vi "Hemolymph.vi"() -> ()   [LabVIEW 2017]
uses:
  <vilib>/vision/NI_Vision_Development_Module.lvlib
panel:
  in  "Tab Control":enum32{"Parameters", "Data"}(tab)
  in  "End":dbl
  in  "Start":dbl
  in  "FPS":dbl
  in  "JPG or AVI":bool
  in  "Frame":i32(slide) min=0 max=10556 step=1 scale=0.0..10556.0
  out "Original":T1(plugin-control)
  in  "Stop Button":bool
  in  "Parameters":T2={"Look for"=0, "Window Size(32x32)"={"SizeX"=32, "SizeY"=32}, "Niblack Deviation Factor"=0.2, "Range"={"Lower value"=128, "Upper value"=255}, "Number of Erosion"=2} {"Range"."Upper value" scale=0.0..255.0; "Range"."Lower value" scale=0.0..255.0; "Niblack Deviation Factor" min=0.0 max=1.0 format="%.2f"; "Window Size(32x32)"."SizeY" min=3 step=1; "Window Size(32x32)"."SizeX" min=3 step=1; "Look for" items=["Bright Objects", "Dark Objects"]}
  in  "Method":i32(ring) items=["Niblack", "Background Correction", "Constant Threshold", "Auto Threshold"]
  out "Threshold":T1(plugin-control)
  out "Improved Threshold":T1(plugin-control)
  out "Clamped":T1(plugin-control)
  in  "Extract Length":bool
  out "Time":dbl[](array[numeric])
  out "Number of frames":dbl
  in  "Fit Length":bool
  out "Velocity":cluster{"Time":dbl[], dbl[]}(graph)
  out "Length":cluster{dbl[], sgl[]}(graph)
  out "Fit":cluster{"Time":dbl[], "mean":dbl[]}[](graph)
  in  "No of Avg":i32
  out "Distance":sgl[](array[numeric]) format="%.2f"
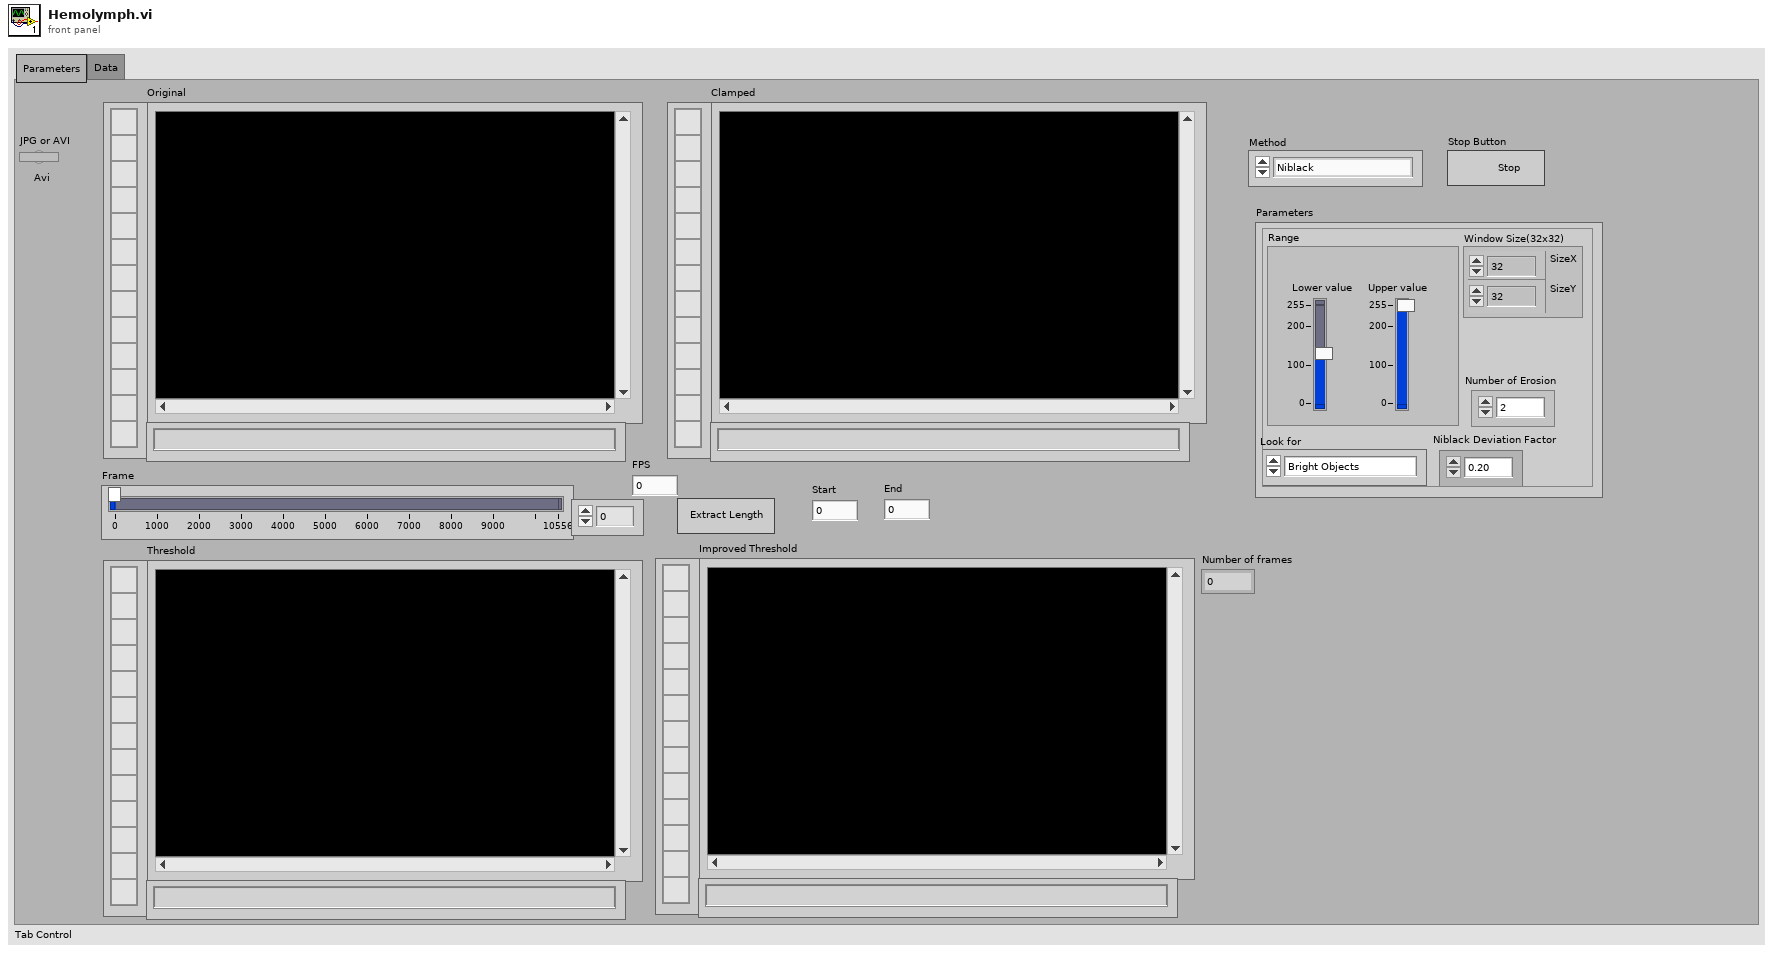
[diagram p1: front panel]
types:
  T1 = typedef "IMAQ Image.ctl" = refnum<image>
  T2 = cluster{"Look for":i32, "Window Size(32x32)":cluster{"SizeX":i32, "SizeY":i32}, "Niblack Deviation Factor":dbl, "Range":cluster{"Lower value":i32, "Upper value":i32}, "Number of Erosion":i32}
  T3 = cluster{"Global Rectangle":i32[], "Contours":cluster{"Contour Type":u32, "ROI Type":u32, "Points":i32[]}[]}
  T4 = typedef "IMAQ Rectangle" = cluster{"Left":i32, "Top":i32, "Right":i32, "Bottom":i32, "Rotation":dbl}
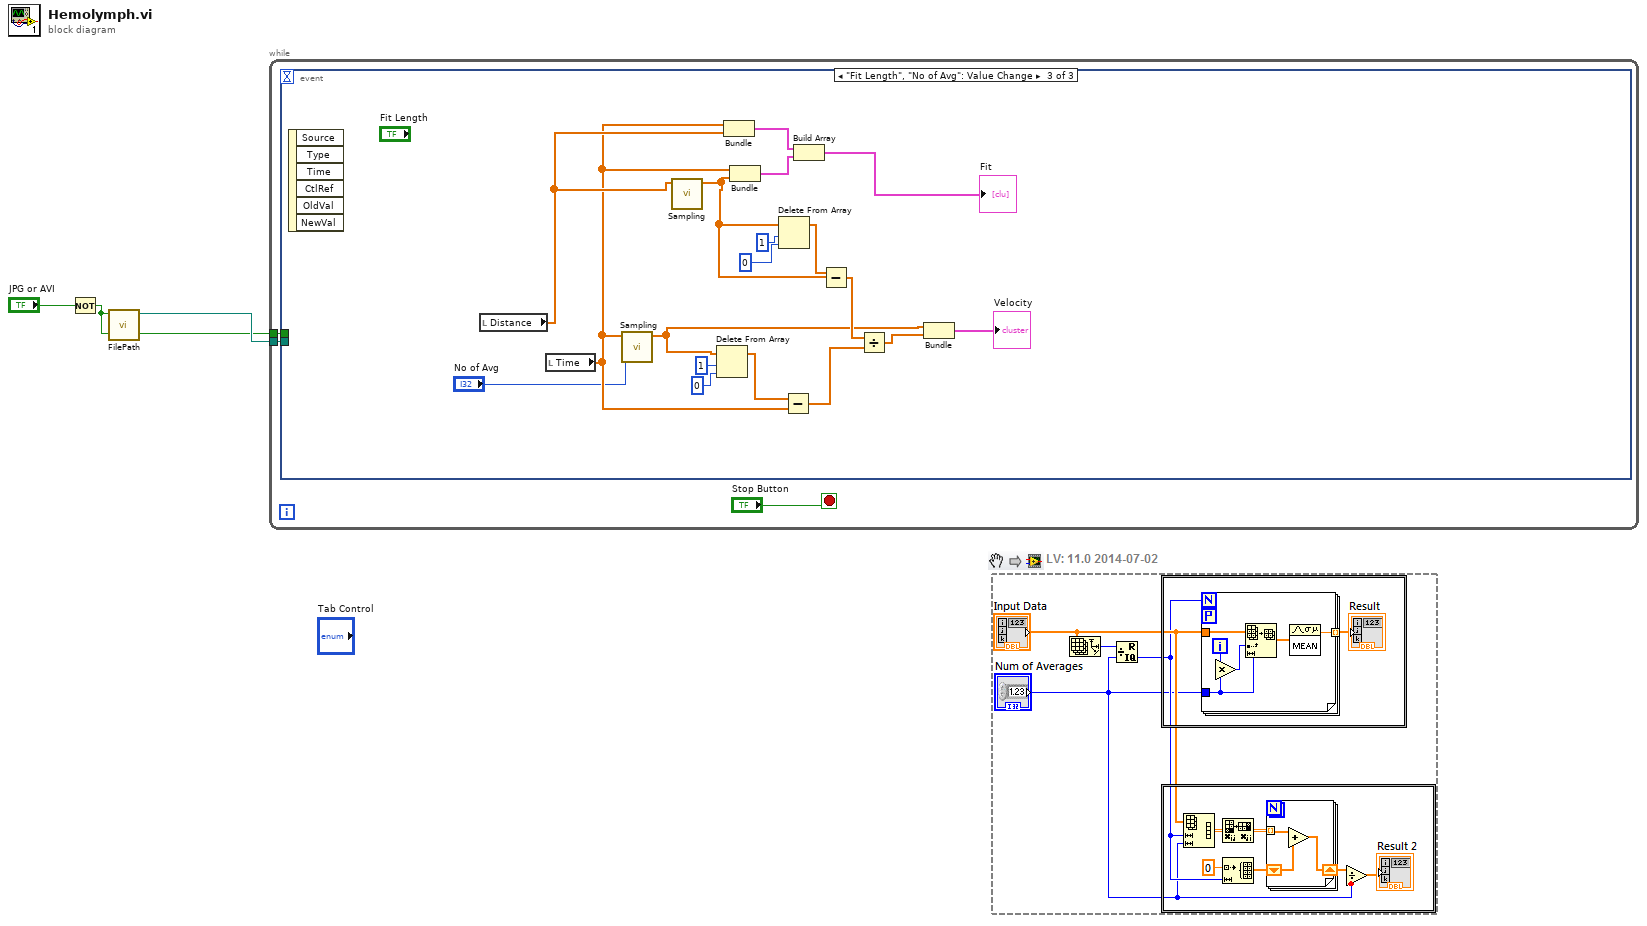
[diagram p0: block diagram]
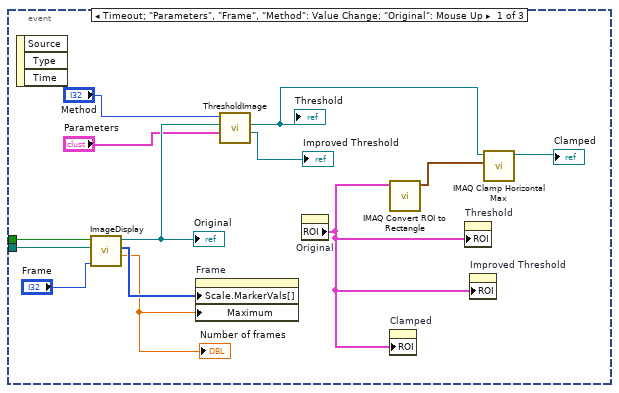
[diagram p2: hidden frame]
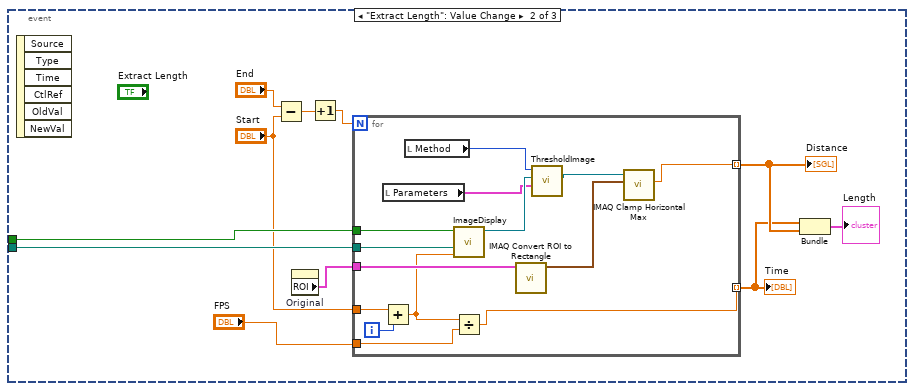
[diagram p3: hidden frame]
diagram:
  n1 = Not(x="JPG or AVI") -> (.not. x?=w1:bool)
  n2 = call "FilePath.vi"("Boolean"=w1) -> ("Path"=w3:path)  [unwired: 10 in]
  n3 = while {
    tunnel: w3 -> [w6]
    tunnel: w1 -> [w5]
    stop <- "Stop Button" stop-if-true
    n4 = event shown="[2] \"Fit Length\", \"No of Avg\": Value Change" {
      selector: _ -> [_ _ _]
      dyn-events: _ -> [_ _ _]
      timeout: _ -> [_ _ _]
      tunnel: w6 -> [w19 w29 _]
      tunnel: w5 -> [w17 w30 _]
      event Timeout; "Parameters", "Frame", "Method": Value Change; "Original": Mouse Up {
        n5 = event-data() -> ()  [unwired: 1 in, 3 out]
        n6 = call "ImageDisplay.vi"("Frame"="Frame", "Path"=w19, "JPG or AVI"=w17) -> ("Number of frames"=w15:dbl, "Frames"=w16:u32[], "Image"=w14:T1)  [unwired: 5 in]
        "Original" <- w14
        "Number of frames" <- w15
        n7 = property on="Frame" class="Slide (strict)"("Scale.MarkerVals[]"=w16, "Maximum"=w15) -> ()  [unwired: 2 in, 2 out]
        n8 = call "ThresholdImage.vi"("Method"="Method", "Image Src"=w14, "Cluster"="Parameters") -> ("Threshold"=w9:T1, "Improved Threshold"=→"Improved Threshold":T1)  [unwired: 6 in]
        "Threshold" <- w9
        n9 = property on="Original" class="ImageControl"() -> ("ROI"=w7:T3)  [unwired: 2 in, 2 out]
        n10 = call "IMAQ Convert ROI to Rectangle"("ROI Descriptor"=w7) -> ("Rectangle"=w10:T4)  [unwired: 8 in, 1 out]
        n11 = property on="Clamped" class="ImageControl"("ROI"=w7) -> ()  [unwired: 2 in, 2 out]
        n12 = property on="Threshold" class="ImageControl"("ROI"=w7) -> ()  [unwired: 2 in, 2 out]
        n13 = property on="Improved Threshold" class="ImageControl"("ROI"=w7) -> ()  [unwired: 2 in, 2 out]
        n14 = call "IMAQ Clamp Horizontal Max"("Rectangle"=w10, "Image"=w9) -> ("Image Out"=→"Clamped":T1)  [unwired: 5 in, 4 out]
      }
      event "Extract Length": Value Change {
        n15 = event-data() -> ()  [unwired: 1 in, 6 out]
        n16 = Subtract(x="End", y="Start") -> (x-y=w25:dbl)
        n17 = property on="Original" class="ImageControl"() -> ("ROI"=w28:T3)  [unwired: 2 in, 2 out]
        n18 = Increment(x=w25) -> (x+1=w24:dbl)
        n19 = for {
          N: w24 -> [_]
          tunnel: w30 -> [w44]
          tunnel: w29 -> [w43]
          tunnel: [w42] -> w21 mode=indexing
          tunnel: w28 -> [w41]
          tunnel: [w39] -> w22 mode=indexing
          tunnel: "FPS" -> [w34]
          tunnel: "Start" -> [w31]
          i -> [w33]
          n20 = local read "Parameters"() -> (w36:T2)
          n21 = Add(x=w31, y=w33) -> (x+y=w32:dbl)
          n22 = local read "Method"() -> (w38:i32)
          n23 = call "ImageDisplay.vi"("Frame"=w32, "Path"=w43, "JPG or AVI"=w44) -> ("Image"=w37:T1)  [unwired: 5 in, 2 out]
          n24 = Divide(x=w32, y=w34) -> (x/y=w42:dbl)
          n25 = call "IMAQ Convert ROI to Rectangle"("ROI Descriptor"=w41) -> ("Rectangle"=w40:T4)  [unwired: 8 in, 1 out]
          n26 = call "ThresholdImage.vi"("Method"=w38, "Image Src"=w37, "Cluster"=w36) -> ("Threshold"=w35:T1)  [unwired: 6 in, 1 out]
          n27 = call "IMAQ Clamp Horizontal Max"("Rectangle"=w40, "Image"=w35) -> ("Distance"=w39:sgl)  [unwired: 5 in, 4 out]
        }
        "Time" <- w21
        "Distance" <- w22
        n28 = Bundle(w21, w22) -> (→"Length":cluster{dbl[], sgl[]})  [unwired: 1 in]
      }
      event "Fit Length", "No of Avg": Value Change {
        n29 = event-data() -> ()  [unwired: 1 in, 6 out]
        n30 = local read "Distance"() -> (w49:sgl[])
        n31 = local read "Time"() -> (w48:dbl[])
        n32 = call "Sampling.vi"("No of Avg"="No of Avg", "Unsampled"=w48) -> ("mean"=w46:dbl[])  [unwired: 8 in, 1 out]
        n33 = call "Sampling.vi"("Unsampled"=w49) -> ("mean"=w45:dbl[])  [unwired: 9 in, 1 out]
        n34 = Delete From Array(array=w46, length=1, index=0) -> (array with subset deleted=w61:dbl[])  [unwired: 1 out]
        n35 = Bundle("Time"=w48, "Distance"=w49) -> (w51:cluster{"Time":dbl[], "Distance":sgl[]})  [unwired: 1 in]
        n36 = Bundle("Time"=w48, "mean"=w45) -> (w52:cluster{"Time":dbl[], "mean":dbl[]})  [unwired: 1 in]
        n37 = Delete From Array(array=w45, length=1, index=0) -> (array with subset deleted=w62:dbl[])  [unwired: 1 out]
        n38 = Subtract(x=w61, y=w48) -> (x-y=w58:dbl[])
        n39 = Build Array(w51, w52) -> (→"Fit":cluster{"Time":dbl[], "mean":dbl[]}[])
        n40 = Subtract(x=w62, y=w45) -> (x-y=w59:dbl[])
        n41 = Divide(x=w59, y=w58) -> (x/y=w57:dbl[])
        n42 = Bundle("mean"=w46, w57) -> (→"Velocity":cluster{"mean":dbl[], dbl[]})  [unwired: 1 in]
      }
    }
  }
